vi "NR Fetch ModAcc.vi"(0 "RFmx Handle In":refnum<k21>, 1 "Selector String":string, 11 "error in (no error)":errorcluster) -> (4 "RFmx Handle Out":refnum<k21>, 6 "ModAcc Results":T1, 15 "error out":errorcluster)   [LabVIEW 2019, in "RFmxNR.lvlib"]
doc: "Fetches common results from the ModAcc measurement."
uses:
  RFmxNR.lvlib
  Typedefs/NR ModAcc Results.ctl
  Typedefs/NR ModAcc Component Carrier Results.ctl
  <resource>/objmgr/RFmxNR.rc
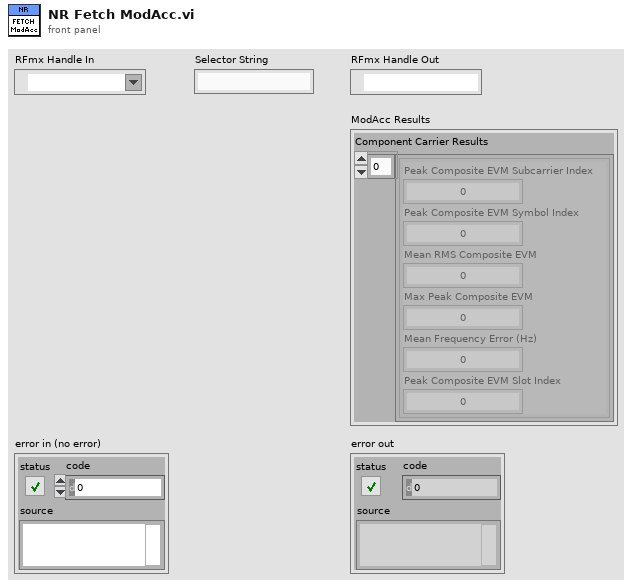
[diagram p1: front panel]
types:
  T1 = typedef "RFmxNR.lvlib/NR ModAcc Results.ctl" = cluster{"Component Carrier Results":T2[]}
  T2 = typedef "RFmxNR.lvlib/NR ModAcc Component Carrier Results.ctl" = cluster{"Peak Composite EVM Subcarrier Index":i32, "Peak Composite EVM Symbol Index":i32, "Mean RMS Composite EVM":dbl, "Max Peak Composite EVM":dbl, "Mean Frequency Error (Hz)":dbl, "Peak Composite EVM Slot Index":i32}
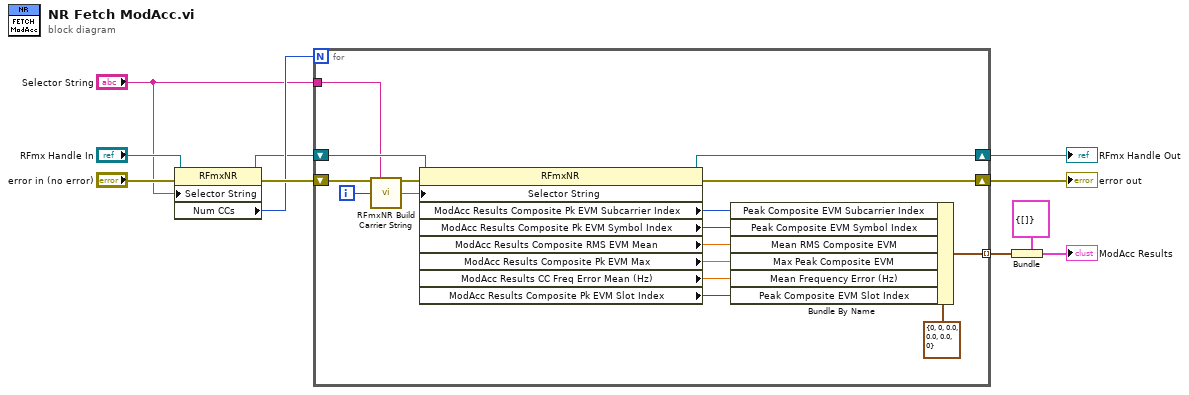
[diagram p0: block diagram]
diagram:
  n1 = property class="RFmxNR"(reference="RFmx Handle In", error in="error in (no error)", "Selector String"="Selector String") -> (reference out=w6:refnum<k21>, error out=w9:errorcluster, "Num CCs"=w8:i32)
  n2 = for {
    N: w8 -> [_]
    tunnel: "Selector String" -> [w14]
    shift-right: [w25] -> w7
    shift-left: w6 -> [w24]
    shift-right: [w23] -> w5
    shift-left: w9 -> [w26]
    tunnel: [w15] -> w3 mode=indexing
    i -> [w12]
    n3 = call <vilib>:"RFmxNR Build Carrier String.vi"("Selector String"=w14, "Carrier Number"=w12) -> ("Selector String Out"=w13:string)  [unwired: 13 in]
    n4 = property class="RFmxNR"(reference=w24, error in=w26, "Selector String"=w13) -> (reference out=w25:refnum<k21>, error out=w23:errorcluster, "ModAcc Results Composite Pk EVM Subcarrier Index"=w21:i32, "ModAcc Results Composite Pk EVM Symbol Index"=w20:i32, "ModAcc Results Composite RMS EVM Mean"=w19:dbl, "ModAcc Results Composite Pk EVM Max"=w18:dbl, "ModAcc Results CC Freq Error Mean (Hz)"=w17:dbl, "ModAcc Results Composite Pk EVM Slot Index"=w16:i32)
    n5 = Bundle By Name(cluster=T2 {"Peak Composite EVM Subcarrier Index"=0, "Peak Composite EVM Symbol Index"=0, "Mean RMS Composite EVM"=0.0, "Max Peak Composite EVM"=0.0, "Mean Frequency Error (Hz)"=0.0, "Peak Composite EVM Slot Index"=0} ("NR ModAcc Component Carrier Results"), "Peak Composite EVM Subcarrier Index"=w21, "Peak Composite EVM Symbol Index"=w20, "Mean RMS Composite EVM"=w19, "Max Peak Composite EVM"=w18, "Mean Frequency Error (Hz)"=w17, "Peak Composite EVM Slot Index"=w16) -> (w15:T2)
  }
  "error out" <- w5
  "RFmx Handle Out" <- w7
  n6 = Bundle(cluster=T1 {"Component Carrier Results"=[]} ("NR ModAcc Results"), "Component Carrier Results"=w3) -> (→"ModAcc Results":T1)
